vi "MH_SetAllChannels.vi"(9 "MH_UIThread_Data":T1 {"Acquisitions" min=0 max=100000000 step=1; "T2 Coincidence Cluster"."Stdev" format="%0.2f"; "T2 Coincidence Cluster"."Mean" format="%0.2f"; "Mode" items=["HIST"=0, "T2"=2, "T3"=3]; "SyncDeadTime" min=800 max=160000 step=1; "SyncEdge" items=["falling", "rising"]; "SyncDivider" items=["1", "2", "4", "8", "16"]; "SyncOffset" min=0 max=100000 step=1; "SyncLevel" min=0 max=800 step=1; "AcqTime" min=1 max=360000 step=1; "Binning" items=["1", "2", "4", "8", "16", "32", "64", "128", "256", "512", "1024", "2048", "4096", "8192", "16384", "32768", "65536", "131072", "262144", "524288", "1048576", "2097152", "4194304", "8388608", "16777216", "3355443225"]; "HistoOffset" min=0 max=500 step=1; "HistoLen" min=1024 max=65536 step=1024; "Channels"."DeadTime" min=800 max=160000 step=1; "Channels"."Edge" items=["falling", "rising"]; "Channels"."Offset" min=-100000 max=100000 step=10; "Channels"."Level" min=-1200 max=1200 step=1}, 10 "AllChannels":T7={"Enable"=TRUE, "Offset"=0, "Level"=20, "Edge"=0, "DeadTime"=1000, "UseDeadTime"=FALSE, "SetEnableAllChan"=TRUE, "SetEdgeAllChan"=TRUE, "SetLevelAllChan"=TRUE, "SetOffsetAllChan"=TRUE, "SetUseDTAllChan"=TRUE, "SetDeadTAllChan"=TRUE} {"DeadTime" min=800 max=160000 step=1; "Edge" items=["falling", "rising"]; "Offset" min=-100000 max=100000 step=10; "Level" min=-1200 max=1200 step=1}, 11 "Channels in":T3[](array[typedef]) {"DeadTime" min=800 max=160000 step=1; "Edge" items=["falling", "rising"]; "Offset" min=-100000 max=100000 step=10; "Level" min=-1200 max=1200 step=1}) -> (2 "MH_UIThread_Data":T1={"Init Info"={"Library Version"="", "Serial No."="", "Model"="", "Partnum"="", "Version"="", "features"=0, "nchannels"=0, "Base Resolution"=0.0, "Bin Steps"=0}, "DevIdx"=0, "SyncDivider"=1, "SyncOffset"=0, "SyncLevel"=50, "Channels"=[], "CurrentChannels"=[], "AcqTime"=1, "Binning"=1, "HistoOffset"=1, "HistoLen"=1024, "StopOvl."=FALSE, "OvlLevel"=1024, "SyncEdge"=1, "StartMeas"=FALSE, "HistoLength"=0, "Resolution"=0.0, "Run cont."=FALSE, "Status"="", "SyncRate"=0, "BitShift"=0, "HistoAcqTime"=0.0, "SyncRateStart"=0, "UseDeadTime"=FALSE, "SyncDeadTime"=800, "SetInpChan"=[], "max value"=[], "CoincidenceArray"=[], "Histo On"=FALSE, "Mode"=0, "Scanning"=FALSE, "Last Move"=FALSE, "Coincidence Window"=0.0, "Max Triggers"=0, "Coincidence Delays"=[], "T2 Coincidences Array"=[], "Clear Graph"=FALSE, "File Save Path"=path "", "T2 Coincidence Cluster"={"Coincidences"=[], "Mean"=[], "Sqrt(mean)"=[], "Stdev"=[]}, "Acquisitions"=0, "HR Array"=[], "Ext. Scanning"=FALSE, "AllanVariance"=[]} {"Acquisitions" min=0 max=100000000 step=1; "T2 Coincidence Cluster"."Stdev" format="%0.2f"; "T2 Coincidence Cluster"."Mean" format="%0.2f"; "Mode" items=["HIST"=0, "T2"=2, "T3"=3]; "SyncDeadTime" min=800 max=160000 step=1; "SyncEdge" items=["falling", "rising"]; "SyncDivider" items=["1", "2", "4", "8", "16"]; "SyncOffset" min=0 max=100000 step=1; "SyncLevel" min=0 max=800 step=1; "AcqTime" min=1 max=360000 step=1; "Binning" items=["1", "2", "4", "8", "16", "32", "64", "128", "256", "512", "1024", "2048", "4096", "8192", "16384", "32768", "65536", "131072", "262144", "524288", "1048576", "2097152", "4194304", "8388608", "16777216", "3355443225"]; "HistoOffset" min=0 max=500 step=1; "HistoLen" min=1024 max=65536 step=1024; "Channels"."DeadTime" min=800 max=160000 step=1; "Channels"."Edge" items=["falling", "rising"]; "Channels"."Offset" min=-100000 max=100000 step=10; "Channels"."Level" min=-1200 max=1200 step=1})   [LabVIEW 2023]
uses:
  ConcreteClasses/ConcreteInstrumentClasses/Multiharp/Multiharp/Types/MH_UIThread_Data_SPI.ctl
  ConcreteClasses/ConcreteInstrumentClasses/Multiharp/Multiharp/_lib/PQ/MultiHarp/MH_InitInfo.ctl
  ConcreteClasses/ConcreteInstrumentClasses/Multiharp/Multiharp/Types/MH_InputChannel.ctl
  ConcreteClasses/ConcreteInstrumentClasses/Multiharp/Multiharp/Types/MH_SetInpChanData.ctl
  ConcreteClasses/ConcreteInstrumentClasses/Multiharp/Multiharp/Types/MH_SetInpChanCmds.ctl
  ConcreteClasses/ConcreteInstrumentClasses/Multiharp/Multiharp/_lib/PQ/MultiHarp/MH_MeasMode.ctl
  typedefs/typedefs.lvlib
panel:
  # "Sync"
  # "Histogram"
  # "Sync"
  # "Histogram"
  # "All Channels"
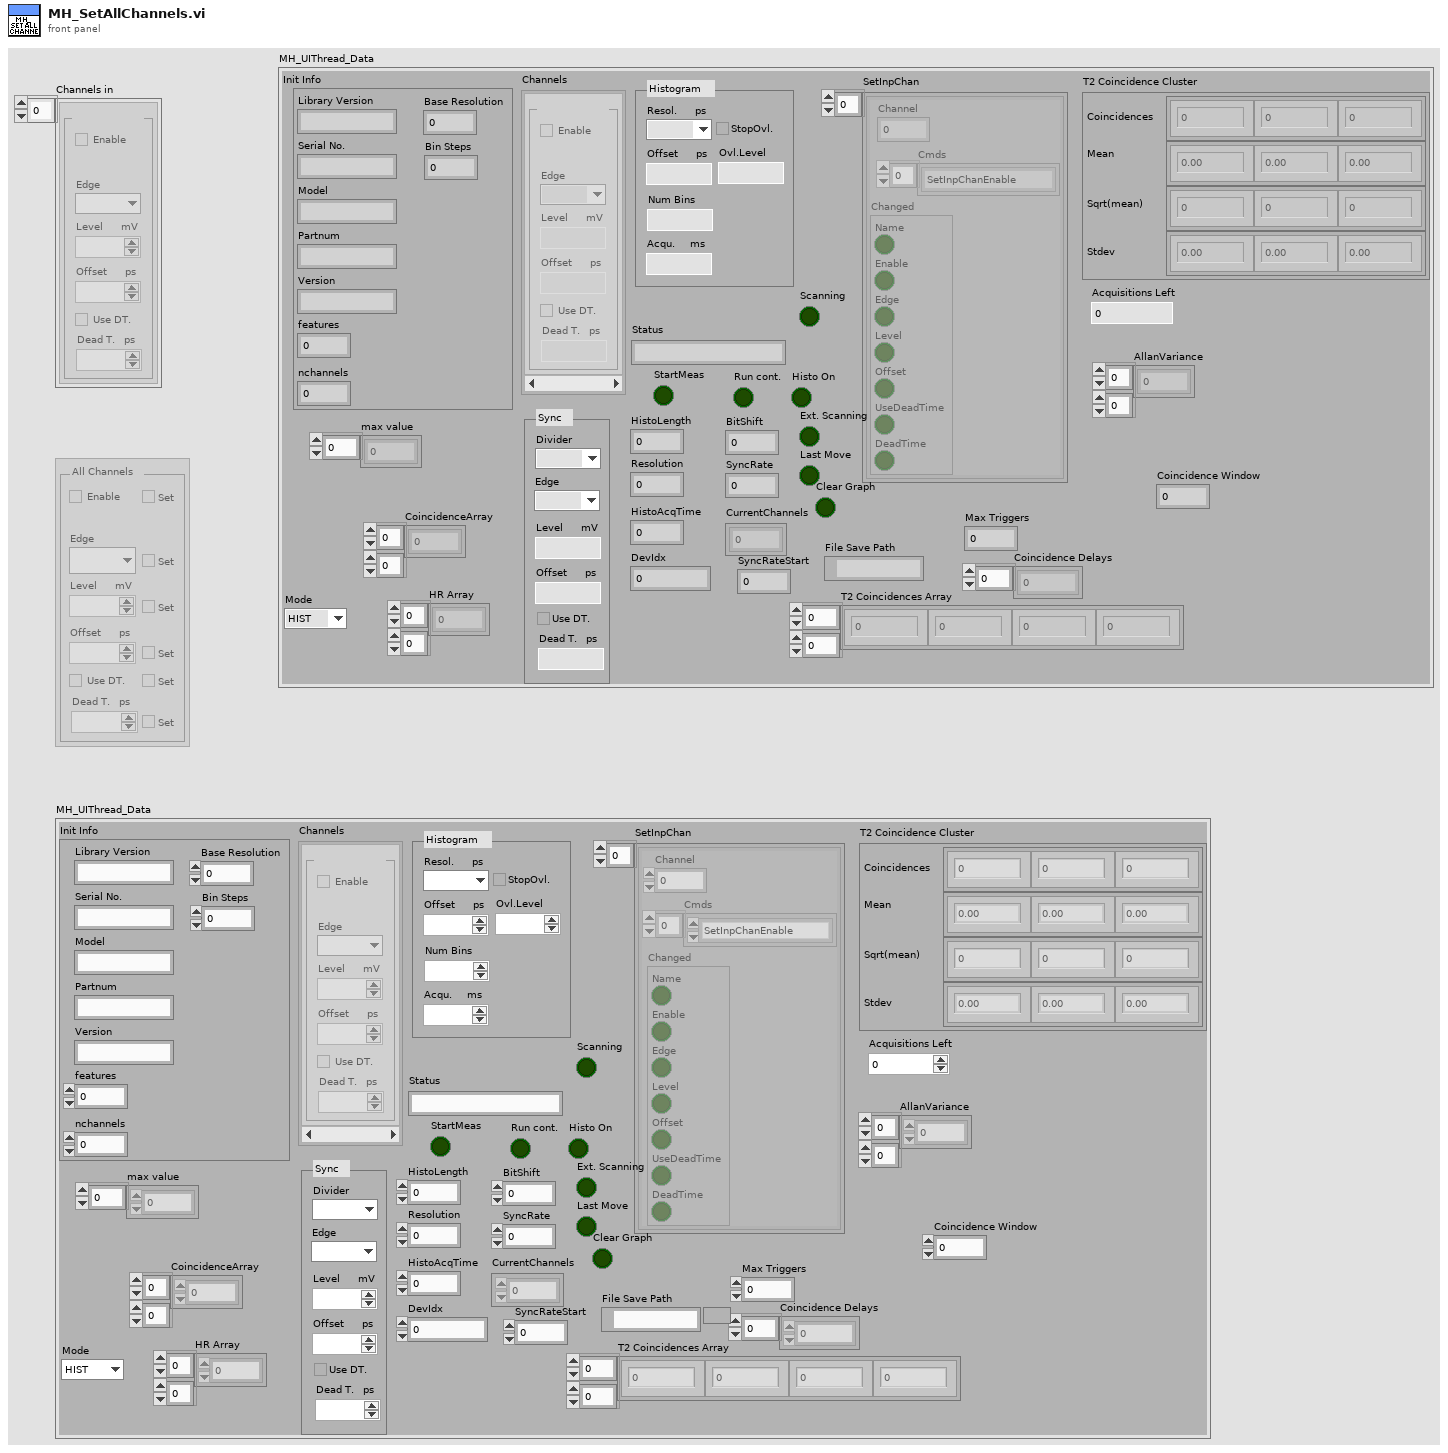
[diagram p1: front panel]
types:
  T1 = typedef "MH_UIThread_Data_SPI.ctl" = cluster{"Init Info":T2, "DevIdx":i32, "SyncDivider":i32, "SyncOffset":i32, "SyncLevel":i32, "Channels":T3[], "CurrentChannels":i32[], "AcqTime":i32, "Binning":i32, "HistoOffset":i32, "HistoLen":i32, "StopOvl.":bool, "OvlLevel":u32, "SyncEdge":i32, "StartMeas":bool, "HistoLength":i32, "Resolution":dbl, "Run cont.":bool, "Status":string, "SyncRate":i32, "BitShift":i32, "HistoAcqTime":dbl, "SyncRateStart":i32, "UseDeadTime":bool, "SyncDeadTime":i32, "SetInpChan":T4[], "max value":u32[], "CoincidenceArray":u32[][], "Histo On":bool, "Mode":T6, "Scanning":bool, "Last Move":bool, "Coincidence Window":dbl, "Max Triggers":i32, "Coincidence Delays":dbl[], "T2 Coincidences Array":i32[][], "Clear Graph":bool, "File Save Path":path, "T2 Coincidence Cluster":cluster{"Coincidences":u32[], "Mean":dbl[], "Sqrt(mean)":dbl[], "Stdev":dbl[]}, "Acquisitions":i32, "HR Array":sgl[][], "Ext. Scanning":bool, "AllanVariance":dbl[][]}
  T2 = typedef "typedefs.lvlib/MH_InitInfo.ctl" = cluster{"Library Version":string, "Serial No.":string, "Model":string, "Partnum":string, "Version":string, "features":i32, "nchannels":i32, "Base Resolution":dbl, "Bin Steps":i32}
  T3 = typedef "MH_InputChannel.ctl" = cluster{"Name":string, "Enable":bool, "Edge":i32, "Level":i32, "Offset":i32, "UseDeadTime":bool, "DeadTime":i32}
  T4 = typedef "MH_SetInpChanData.ctl" = cluster{"Channel":i32, "Cmds":T5[], "Changed":cluster{"Name":bool, "Enable":bool, "Edge":bool, "Level":bool, "Offset":bool, "UseDeadTime":bool, "DeadTime":bool}}
  T5 = typedef "MH_SetInpChanCmds.ctl" = enum16{"SetInpChanEnable", "SetInpChanOffset", "SetInpChanDeadTime", "SetInpChanTrg"}
  T6 = typedef "MH_MeasMode.ctl" = i32
  T7 = cluster{"Enable":bool, "Offset":i32, "Level":i32, "Edge":i32, "DeadTime":i32, "UseDeadTime":bool, "SetEnableAllChan":bool, "SetEdgeAllChan":bool, "SetLevelAllChan":bool, "SetOffsetAllChan":bool, "SetUseDTAllChan":bool, "SetDeadTAllChan":bool}
  T8 = typedef "MH_InputChannel2.ctl" = cluster{"Name":string, "Enable":bool, "Edge":i32, "Level":i32, "Offset":i32, "UseDeadTime":bool, "DeadTime":i32}
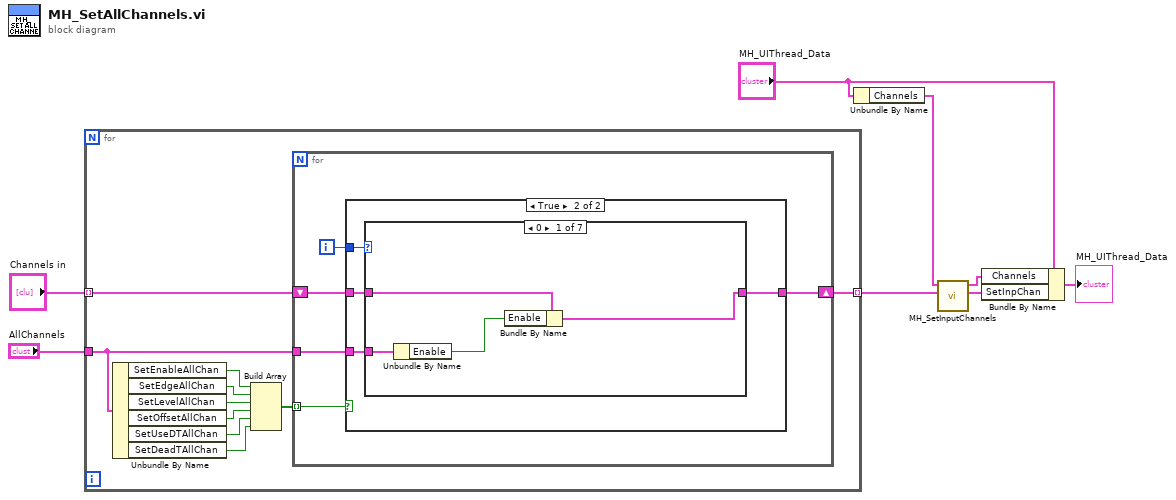
[diagram p0: block diagram]
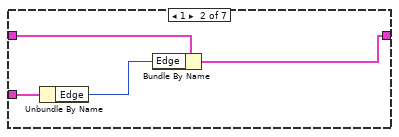
[diagram p3: hidden frame]
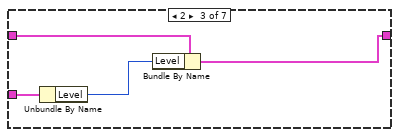
[diagram p4: hidden frame]
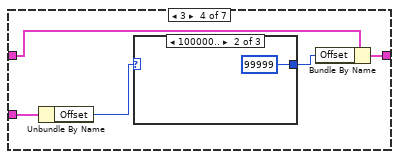
[diagram p5: hidden frame]
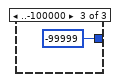
[diagram p7: hidden frame]
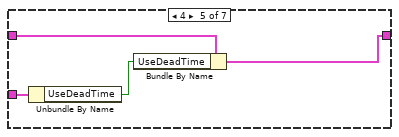
[diagram p8: hidden frame]
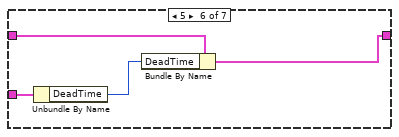
[diagram p9: hidden frame]
diagram:
  n1 = for {
    tunnel: "Channels in" -> [w11] mode=indexing
    tunnel: "AllChannels" -> [w10]
    tunnel: [w9] -> w5 mode=indexing
    n2 = Unbundle By Name(w10) -> ("SetEnableAllChan"=w12:bool, "SetEdgeAllChan"=w13:bool, "SetLevelAllChan"=w14:bool, "SetOffsetAllChan"=w15:bool, "SetUseDTAllChan"=w16:bool, "SetDeadTAllChan"=w17:bool)
    n3 = Build Array(w12, w13, w14, w15, w16, w17) -> (w18:bool[])
    n4 = for {
      tunnel: w18 -> [w23] mode=indexing
      shift-right: [w20] -> w9
      shift-left: w11 -> [w21]
      tunnel: w10 -> [w19]
      i -> [w22]
      n5 = case shown="True" w23 {
        tunnel: w22 -> [_ w28]
        tunnel: w19 -> [_ w27]
        tunnel: w21 -> [w24 w26]
        tunnel: [w24 w25] -> w20
        frame False {
        }
        frame True {
          n6 = case shown="0" w28 {
            tunnel: w27 -> [w32 w36 w40 w45 w52 w56 _]
            tunnel: w26 -> [w31 w35 w39 w44 w51 w55 w57]
            tunnel: [w29 w33 w37 w43 w49 w53 w57] -> w25
            frame 0 {
              n7 = Unbundle By Name(w32) -> ("Enable"=w30:bool)
              n8 = Bundle By Name(cluster=w31, "Enable"=w30) -> (w29:T3)
            }
            frame 1 {
              n9 = Unbundle By Name(w36) -> ("Edge"=w34:i32)
              n10 = Bundle By Name(cluster=w35, "Edge"=w34) -> (w33:T3)
            }
            frame 2 {
              n11 = Unbundle By Name(w40) -> ("Level"=w38:i32)
              n12 = Bundle By Name(cluster=w39, "Level"=w38) -> (w37:T3)
            }
            frame 3 {
              n13 = Unbundle By Name(w45) -> ("Offset"=w42:i32)
              n14 = case shown="100000.." w42 {
                selector: w42 -> [w46 _ _]
                tunnel: [w46 99999 ("SyncOffset") -99999 ("SyncOffset")] -> w41
                frame Default {
                }
                frame 100000.. {
                }
                frame ..-100000 {
                }
              }
              n15 = Bundle By Name(cluster=w44, "Offset"=w41) -> (w43:T3)
            }
            frame 4 {
              n16 = Unbundle By Name(w52) -> ("UseDeadTime"=w50:bool)
              n17 = Bundle By Name(cluster=w51, "UseDeadTime"=w50) -> (w49:T3)
            }
            frame 5 {
              n18 = Unbundle By Name(w56) -> ("DeadTime"=w54:i32)
              n19 = Bundle By Name(cluster=w55, "DeadTime"=w54) -> (w53:T3)
            }
            frame Default {
            }
          }
        }
      }
    }
  }
  n20 = Unbundle By Name("MH_UIThread_Data") -> ("Channels"=w6:T3[])
  n21 = call "MH_SetInputChannels.vi"("Channels new"=w5, "Channels old"=w6) -> ("SetInpChan"=w3:T4[], "Channels"=w4:T8[])  [unwired: 8 in]
  n22 = Bundle By Name(cluster="MH_UIThread_Data", "Channels"=w4, "SetInpChan"=w3) -> (→"MH_UIThread_Data":T1)
